vi "图片格式转换.vi"() -> ()   [LabVIEW 2020]
panel:
  in  "?":bool
  in  "?":bool
  in  "?":bool
  out "?":T1(plugin-control)
  in  "转换类型":enum16{".jpg", ".png", ".bmp", ".tiff", ""}(ring)
  out "error out":errorcluster
  in  "error in (no error)":errorcluster
  in  "文件命名":string
  in  "存储路径":path
  out "文件类型":string
  # "请对以下内容设置完成后再进行转换"
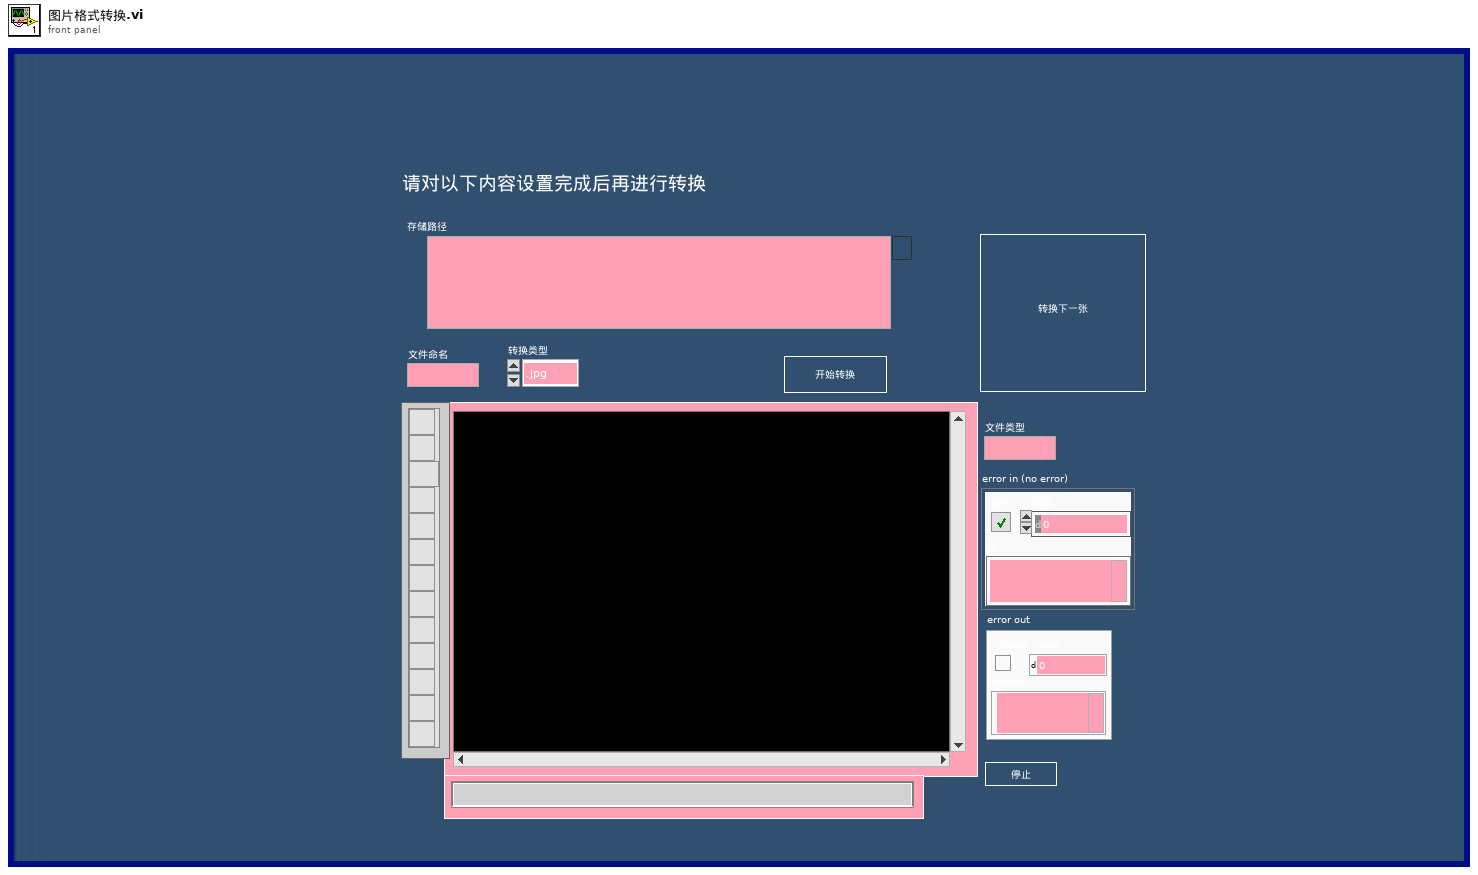
[diagram p1: front panel]
types:
  T1 = typedef "IMAQ Image.ctl" = refnum<image>
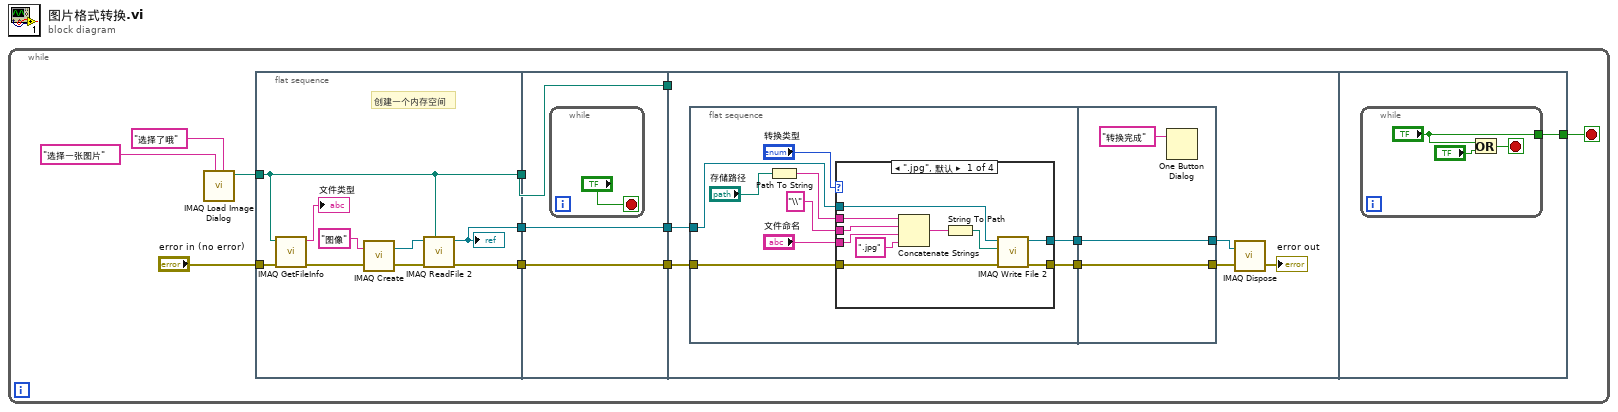
[diagram p0: block diagram]
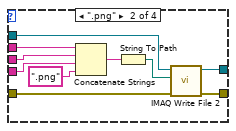
[diagram p2: hidden frame]
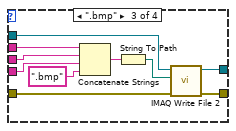
[diagram p3: hidden frame]
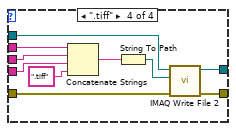
[diagram p4: hidden frame]
diagram:
  n1 = while {
    stop <- w7 stop-if-true
    n2 = call "IMAQ Load Image Dialog"("Button Label"="选择了哦", "Prompt"="选择一张图片") -> ("Path"=w8:path)  [unwired: 7 in, 2 out]
    n3 = flat-sequence {
      tunnel: "error in (no error)" -> [w20]
      tunnel: w8 -> [w13]
      tunnel: [w15] -> w6
      tunnel: [w14] -> w4
      tunnel: [w13] -> w2
      tunnel: w6 -> [w23]
      tunnel: [w23] -> w5
      tunnel: w4 -> [w22]
      tunnel: [w22] -> w3
      tunnel: w2 -> [w21]
      tunnel: [w21] -> w1
      tunnel: w5 -> [w31]
      tunnel: w3 -> [w30]
      tunnel: w1 -> [_]
      tunnel: [w84] -> w7
      frame #0 {
        # "创建一个内存空间"
        n4 = call "IMAQ GetFileInfo"("error in (no error)"=w20, "File Path"=w13) -> ("error out"=w17:errorcluster, "File Type"=→"文件类型":string)  [unwired: 3 in, 5 out]
        n5 = call "IMAQ Create"("Image Name"="图像", "error in (no error)"=w17) -> ("New Image"=w19:T1, "error out"=w16:errorcluster)  [unwired: 3 in]
        n6 = call "IMAQ ReadFile 2"("File Path"=w13, "error in (no error)"=w16, "Image"=w19) -> ("error out"=w15:errorcluster, "Image Out"=w14:T1)  [unwired: 4 in, 3 out]
        "?" <- w14
      }
      frame #1 {
        n7 = while {
          stop <- "?" stop-if-true
        }
      }
      frame #2 {
        n8 = flat-sequence {
          tunnel: w31 -> [w40]
          tunnel: w30 -> [w39]
          tunnel: [w38] -> w26
          tunnel: [w37] -> w25
          tunnel: [w82] -> w27
          tunnel: [w83] -> w29
          tunnel: w26 -> [w83]
          tunnel: w25 -> [w82]
          frame #0 {
            n9 = Path To String(path="存储路径") -> (string=w34:string)
            n10 = case shown="\".jpg\", 默认" "转换类型" {
              tunnel: w40 -> [w48 w60 w69 w79]
              tunnel: w39 -> [w50 w59 w70 w80]
              tunnel: [w47 w58 w67 w77] -> w38
              tunnel: [w49 w57 w68 w78] -> w37
              tunnel: w34 -> [w43 w53 w63 w75]
              tunnel: "\\" ("字符串") -> [w44 w54 w64 w74]
              tunnel: "文件命名" -> [w42 w52 w62 w73]
              frame ".jpg", Default {
                n11 = Concatenate Strings(w43, w44, w42, ".jpg" ("字符串")) -> (w46:string)
                n12 = String To Path(string=w46) -> (path=w41:path)
                n13 = call-poly "IMAQ Write File 2"("error in (no error)"=w48, "File Path"=w41, "Image"=w50) -> ("error out"=w47:errorcluster, "Image Out (duplicate)"=w49:T1)  [unwired: 7 in]
              }
              frame ".png" {
                n14 = Concatenate Strings(w53, w54, w52, ".png" ("字符串")) -> (w56:string)
                n15 = String To Path(string=w56) -> (path=w51:path)
                n16 = call-poly "IMAQ Write File 2"("error in (no error)"=w60, "File Path"=w51, "Image"=w59) -> ("error out"=w58:errorcluster, "Image Out (duplicate)"=w57:T1)  [unwired: 7 in]
              }
              frame ".bmp" {
                n17 = Concatenate Strings(w63, w64, w62, ".bmp" ("字符串")) -> (w66:string)
                n18 = String To Path(string=w66) -> (path=w61:path)
                n19 = call-poly "IMAQ Write File 2"("error in (no error)"=w69, "File Path"=w61, "Image"=w70) -> ("error out"=w67:errorcluster, "Image Out (duplicate)"=w68:T1)  [unwired: 7 in]
              }
              frame ".tiff" {
                n20 = Concatenate Strings(w75, w74, w73, ".tiff" ("字符串")) -> (w76:string)
                n21 = String To Path(string=w76) -> (path=w72:path)
                n22 = call-poly "IMAQ Write File 2"("error in (no error)"=w79, "File Path"=w72, "Image"=w80) -> ("error out"=w77:errorcluster, "Image Out (duplicate)"=w78:T1)  [unwired: 7 in]
              }
            }
          }
          frame #1 {
            n23 = One Button Dialog(message="转换完成" ("消息")) -> ()  [unwired: 1 in, 1 out]
          }
        }
        n24 = call "IMAQ Dispose"("Image"=w27, "error in (no error)"=w29) -> ("error out"=→"error out":errorcluster)  [unwired: 4 in]
      }
      frame #3 {
        n25 = while {
          tunnel: ["?"] -> w84
          stop <- w87 stop-if-true
          n26 = Or(x="?", y="?") -> (x .or. y?=w87:bool)
        }
      }
    }
  }
